vi "New section.vi"(8 "error in (no error)":errorcluster, 10 "Section name":string, 11 "Plain Text Report In":refnum<class "Plain Text Report.lvclass">) -> (0 "error out":errorcluster, 3 "Plain Text Report Out":refnum<class "Plain Text Report.lvclass">)   [LabVIEW 2020, in "Plain Text Report.lvclass"]
uses:
  Plain Text Report.lvclass
  Plain Text Report.lvclass/Plain Text Report.ctl
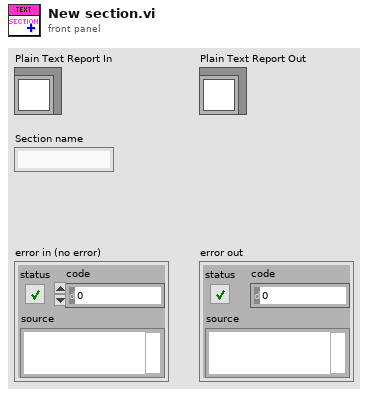
[diagram p1: front panel]
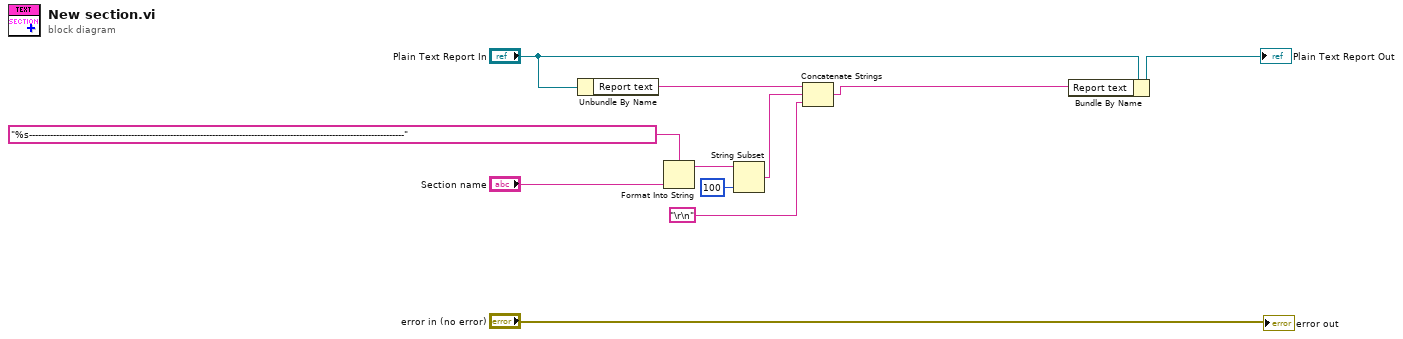
[diagram p0: block diagram]
diagram:
  n1 = Unbundle By Name("Plain Text Report In") -> ("Report text"=w2:string)
  n2 = Format Into String(format string="%s-----------------------------------------------------------------------------------------------------------------------------", "Section name") -> (resulting string=w6:string)  [unwired: 2 in, 1 out]
  n3 = String Subset(string=w6, length (rest)=100 ("length (rest)")) -> (substring=w5:string)  [unwired: 1 in]
  n4 = Concatenate Strings(w2, w5, "\r\n") -> (w1:string)
  n5 = Bundle By Name(cluster="Plain Text Report In", "Report text"=w1) -> (→"Plain Text Report Out":refnum<class "Plain Text Report.lvclass">)
  "error out" <- "error in (no error)"
